vi "Get Timing Results.vi"(8 "error in (no error)":errorcluster, 11 "Execution Profiler in":refnum<class "Execution Profiler.lvclass">) -> (0 "error out":errorcluster, 2 "Timing Results":map{string, dbl}(c390), 3 "Execution Profiler out":refnum<class "Execution Profiler.lvclass">)   [LabVIEW 2020, in "Execution Profiler.lvlib" / "Execution Profiler.lvclass"]
uses:
  Execution Profiler.lvclass
  Execution Profiler.lvclass/Execution Profiler.ctl
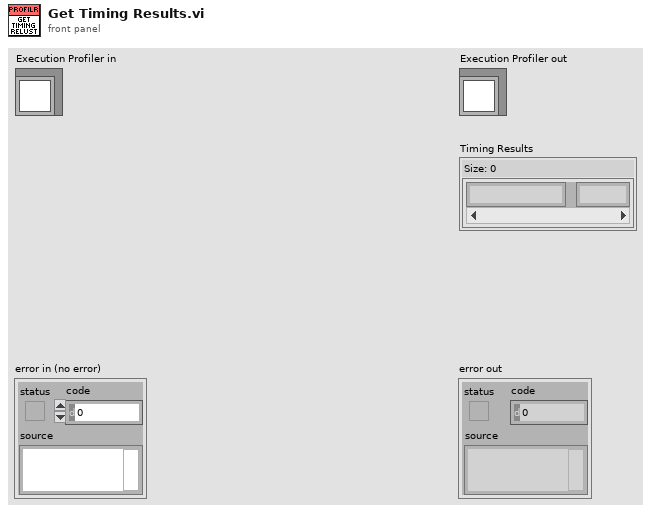
[diagram p1: front panel]
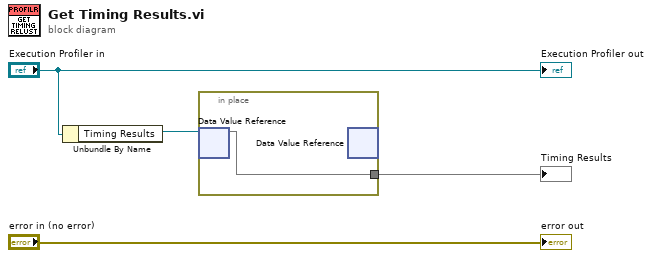
[diagram p0: block diagram]
diagram:
  n1 = Unbundle By Name("Execution Profiler in") -> ("Timing Results"=w2:refnum<data-value>)
  n2 = in-place {
    in-place-border: [w5] -> w1
    n3 = in-place-dvr #1(w2) -> (w5:map{string, dbl})  [unwired: 1 out]
    n4 = in-place-dvr #1() -> ()  [unwired: 1 in, 2 out]
  }
  "Timing Results" <- w1
  "error out" <- "error in (no error)"
  "Execution Profiler out" <- "Execution Profiler in"
